vi "GVmotor_get_Analog.vi"(8 "error in (no error)":errorcluster, 10 "milliseconds to wait":u32=100, 11 "VISA resource name":refnum<visa-resource-name>) -> (0 "error out":errorcluster, 2 "Analog":dbl, 3 "VISA resource name out":refnum<visa-resource-name>)   [LabVIEW 2019]
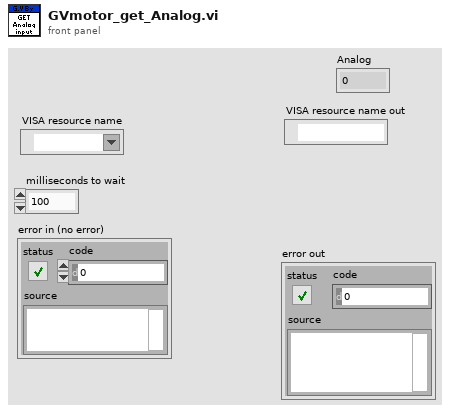
[diagram p1: front panel]
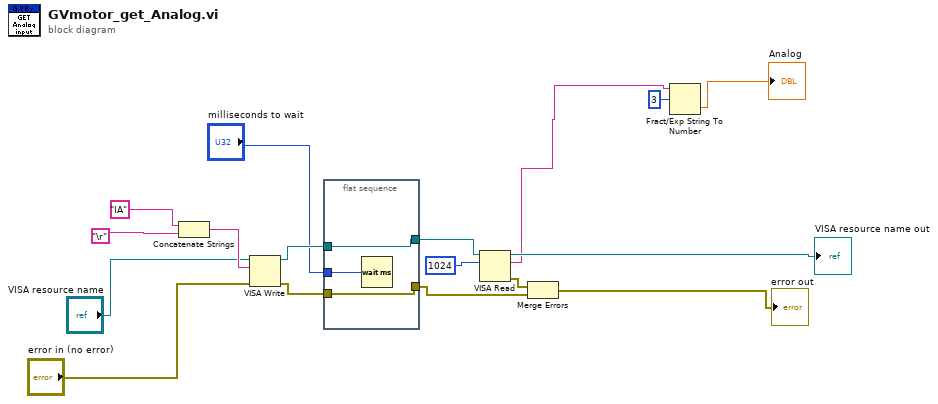
[diagram p0: block diagram]
diagram:
  n1 = Concatenate Strings("IA" ("string"), "\r") -> (w17:string)
  n2 = VISA Write(VISA resource name="VISA resource name", write buffer=w17, error in (no error)="error in (no error)") -> (VISA resource name out=w13:refnum<visa-resource-name>, error out=w14:errorcluster)  [unwired: 1 out]
  n3 = flat-sequence {
    tunnel: [w20] -> w8
    tunnel: w14 -> [w20]
    tunnel: [w19] -> w12
    tunnel: w13 -> [w19]
    tunnel: "milliseconds to wait" -> [w18]
    frame #0 {
      n4 = Wait (ms)(milliseconds to wait=w18) -> ()  [unwired: 1 out]
    }
  }
  n5 = VISA Read(VISA resource name=w12, byte count=u32 1024) -> (VISA resource name out=→"VISA resource name out":refnum<visa-resource-name>, read buffer=w2:string, error out=w7:errorcluster)  [unwired: 1 in, 1 out]
  n6 = Merge Errors(w7, w8) -> (→"error out":errorcluster)
  n7 = Fract/Exp String To Number(string=w2, offset=3) -> (number=→"Analog":dbl)  [unwired: 2 in, 1 out]
